vi "SVT Idle Channel Noise.vi"   [LabVIEW 2017, in "SoundVib_SingleTone.lvlib"]
doc: "Computes idle channel noise, median noise level, and maximum spur of <B>scaled signal</B> and <B>frequency range</B>. This VI also computes the signal-to-noise ratio (SNR) measured without a signal, provided you supply a <B>full-scale level</B>. Wire data to the <B>scaled signal [EU]</B> input to determine the polymorphic instance to use or manually select the instance."
uses:
  <vilib>/addons/Sound and Vibration/svt_Single Tone Measurements/SoundVib_SingleTone.lvlib
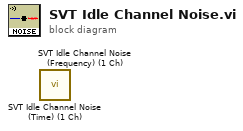
[diagram p0: block diagram]
diagram:
  n1 = call <vilib>:"SVT Idle Channel Noise (Time) (1 Ch).vi"() -> ()  [unwired: 12 in, 8 out]
  n2 = call <vilib>:"SVT Idle Channel Noise (Frequency) (1 Ch).vi"() -> ()  [unwired: 12 in, 8 out]
